vi "Turn.vi"(9 "Gyro Setpoint":dbl, 10 "Turn Right?":bool) -> ()   [LabVIEW 2012]
uses:
  System Set Points and States.vi
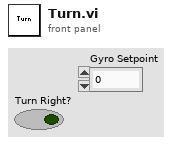
[diagram p1: front panel]
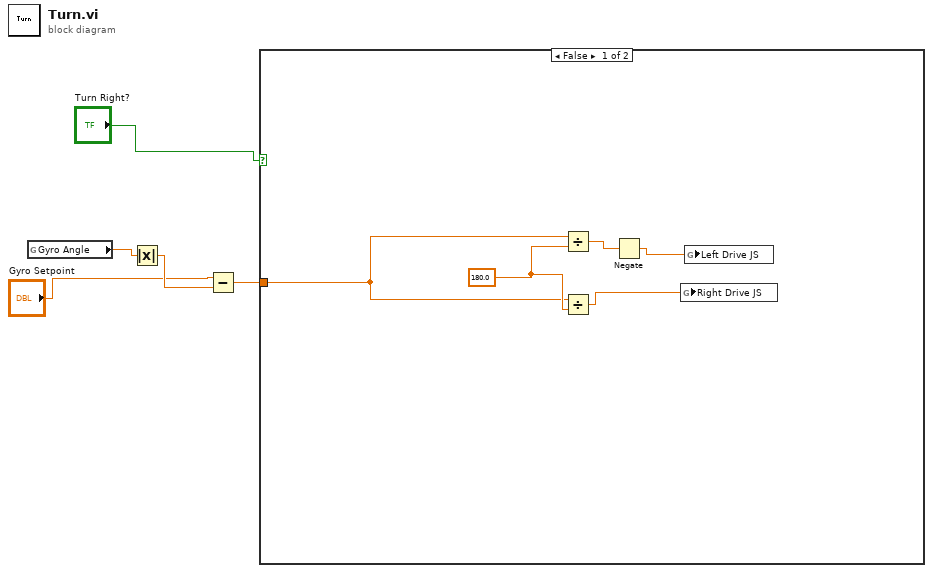
[diagram p0: block diagram]
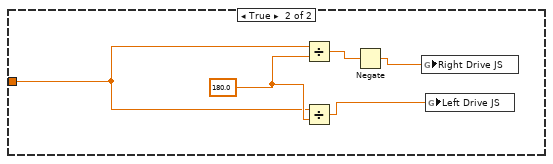
[diagram p2: hidden frame]
diagram:
  n1 = global read "System Set Points and States.vi" "Gyro Angle"() -> (w5:dbl)
  n2 = Absolute Value(x=w5) -> (abs(x)=w4:dbl)
  n3 = Subtract(x="Gyro Setpoint", y=w4) -> (x-y=w3:dbl)
  n4 = case shown="False" "Turn Right?" {
    tunnel: w3 -> [w6 w11]
    frame False {
      w7 = 180.0 ("y")
      n5 = Divide(x=w6, y=w7) -> (x/y=w9:dbl)
      n6 = Divide(x=w6, y=w7) -> (x/y=w10:dbl)
      n7 = Negate(x=w9) -> (-x=w8:dbl)
      n8 = global write "System Set Points and States.vi" "Right Drive JS"(w10) -> ()
      n9 = global write "System Set Points and States.vi" "Left Drive JS"(w8) -> ()
    }
    frame True {
      w12 = 180.0 ("y")
      n10 = Divide(x=w11, y=w12) -> (x/y=w14:dbl)
      n11 = Divide(x=w11, y=w12) -> (x/y=w15:dbl)
      n12 = Negate(x=w14) -> (-x=w13:dbl)
      n13 = global write "System Set Points and States.vi" "Right Drive JS"(w13) -> ()
      n14 = global write "System Set Points and States.vi" "Left Drive JS"(w15) -> ()
    }
  }
